vi "Stop Initiate RUN Procedure.vi"(8 "error in (no error)":errorcluster, 10 "Stop for good":bool, 11 "Tamer in":refnum<class "Tamer.lvclass">) -> (0 "error out":errorcluster, 3 "Tamer out":refnum<class "Tamer.lvclass">)   [LabVIEW 2020, in "TALOS.lvlib" / "Tamer.lvlib" / "Tamer.lvclass"]
uses:
  Tamer.lvclass
  C:/LabVIEW Code/TALOS/talos/Father of all uServices/Father of all uServices/Father of all uServices.lvclass
  Tamer.lvclass/Tamer.ctl
  Tamer Consumer Case Selector.ctl
  Guardian/Guardian/Requests.ctl
  Run Utilities/TypeDefs/Monkey Status.ctl
  Guardian/Guardian Messages/Requests from uServices Msg/Requests from uServices Msg.lvclass/Requests from uServices Msg.ctl
  Ancestor/Ancestor/Ancestor.lvclass/Ancestor.ctl
  Guardian/Guardian Messages/Requests from uServices Msg/Send Requests from uServices.vi
  Support VIs/Generate Error.vi
  FGV/Error Memory/Get Error Description.vi
  Support VIs/Get PC name.vi
  Ancestor/Ancestor/Read ID.vi
  Support VIs/Get Class Name.vi
  <vilib>/Utility/error.llb/Clear Errors.vi
  FGV/Error Memory/Error Memory Core.vi
  <vilib>/AdvancedString/Delimited String to 1D String Array.vi
  Support VIs/Circus Root Path.vi
  FGV/Error Memory/Error Crt Lvl checker.vi
  FGV/Error Memory/Error Memory Core.vi/40c8088d-b597-4017-91af-faa98e00292e.vi
  FGV/Error Memory/Error Memory Core.vi/d4a3ab98-063c-4e44-b43d-fbdcfe6c2be2.vi
  Father of all uServices/Father of all uServices/Father of all uServices.lvclass
  C:/LabVIEW Code/TALOS/builds/Actor Framework PPL/Actor Framework.lvlibp/1abvi3w/vi.lib/ActorFramework/Actor/Actor.lvclass
  builds/Actor Framework PPL/Actor Framework.lvlibp/1abvi3w/vi.lib/ActorFramework/Actor/Read Caller Enqueuer.vi
  builds/Actor Framework PPL/Actor Framework.lvlibp/1abvi3w/vi.lib/ActorFramework/Message Enqueuer/Enqueue.vi
  Support VIs/Global Memory.vi
  <vilib>/Utility/LVClass/Get LV Class Name.vi
  Support VIs/Is in Packed Library.vi
  Support VIs/TALOS Root path.vi
  Support VIs/Read CSV worksheet.vi
  Support VIs/Global Constants.vi
  <vilib>/Utility/error.llb/General Error Handler.vi
  Support VIs/Error Log.vi
  Guardian/Guardian Messages/Requests from uServices Msg/Requests from uServices Msg.lvclass
  Ancestor/Ancestor/Ancestor.lvclass
  <vilib>/Comparison/Equal/Equal Functor/Equal Functor.lvclass
  TALOS.lvlib
  Guardian/Guardian/Guardian.lvclass
  Run Utilities/Run Utilities.lvlib
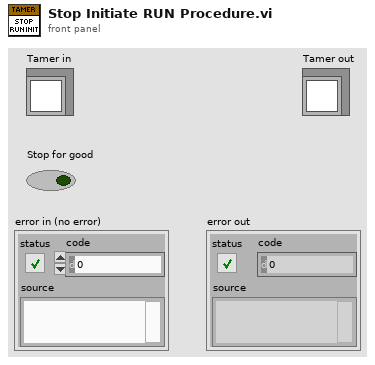
[diagram p1: front panel]
types:
  T1 = typedef "TALOS.lvlib/Tamer.lvlib/Tamer.lvclass/Tamer Consumer Case Selector.ctl" = enum16{"New schedule", "Initiate RUN", "Parse Schedules", "Script Checker", "Banana after Quality Check", "Update Crit Lvl", "Propagate Banana", "Reply from Guardian", "Reply from uService", "Timeout of RUN", "uService Replies Check", "Update from Monkey", "Monkey Died", "Reschedule", "Rerun", "Stop DAQ", "Stop Schedule", "Skip Run", "Kill Process", "Update GV"}
  T2 = typedef "TALOS.lvlib/Run Utilities.lvlib/Monkey Status.ctl" = enum16{"Init", "Paused", "Ongoing", "Stopped", "Finished (no errors)", "Finished (with errors)"}
  T3 = typedef "TALOS.lvlib/Guardian.lvlib/Guardian.lvclass/Requests.ctl" = enum16{"Ready to Launch", "Start RUN", "Stop RUN", "Update DAQ Params", "Update Error Listbox", "Update Run Status", "Update Kasli Log", "Run Stopped with Errors", "Switch uS View"}
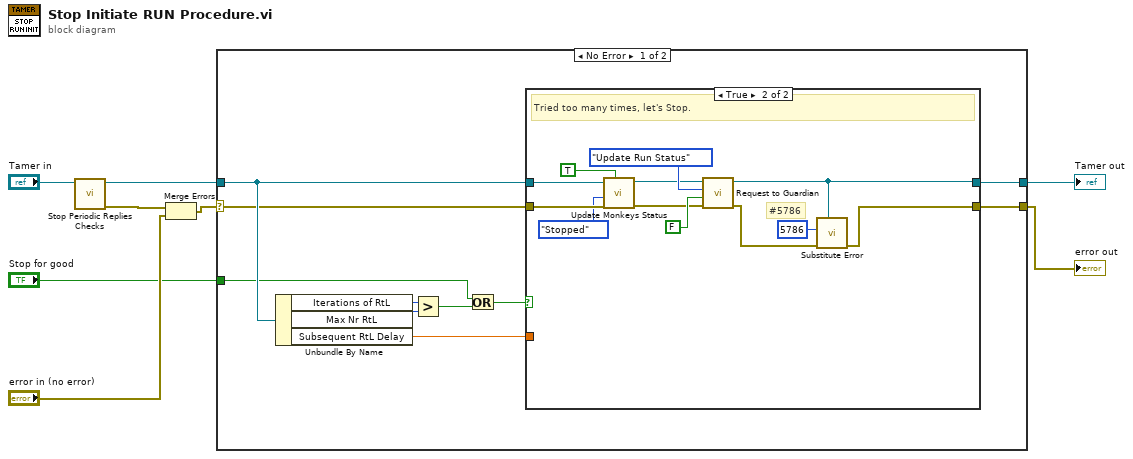
[diagram p0: block diagram]
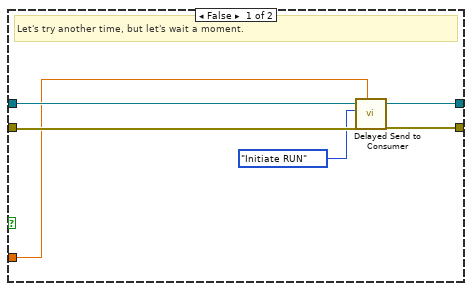
[diagram p2: hidden frame]
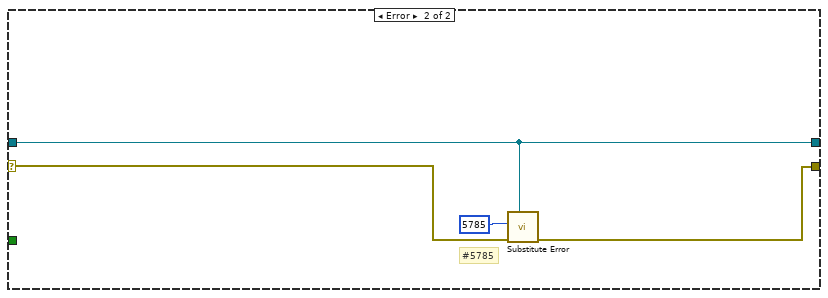
[diagram p3: hidden frame]
diagram:
  n1 = call-dynamic "Stop Periodic Replies Checks.vi"("Tamer in"="Tamer in") -> ("error out"=w2:errorcluster, "Tamer out"=w3:refnum<class "Tamer.lvclass">)  [unwired: 9 in]
  n2 = Merge Errors(w2, "error in (no error)") -> (w5:errorcluster)
  n3 = case shown="No Error" w5 {
    selector: w5 -> [w15 w37]
    tunnel: w3 -> [w17 w38]
    tunnel: [w16 w38] -> w6
    tunnel: [w14 w40] -> w8
    tunnel: "Stop for good" -> [w11 _]
    frame No Error {
      n4 = Unbundle By Name(w17) -> ("Iterations of RtL"=w18:u8, "Max Nr RtL"=w10:u8, "Subsequent RtL Delay"=w9:dbl)
      n5 = Greater?(x=w18, y=w10) -> (0:w13:bool)
      n6 = Or(x=w11, y=w13) -> (x .or. y?=w12:bool)
      n7 = case shown="True" w12 {
        tunnel: w17 -> [w24 w30]
        tunnel: [w23 w34] -> w16
        tunnel: w15 -> [w21 w28]
        tunnel: [w22 w36] -> w14
        tunnel: w9 -> [w20 _]
        frame False {
          # "Let's try another time, but let's wait a moment."
          n8 = call "Delayed Send to Consumer.vi"("Seconds (5)"=w20, "error in (no error)"=w21, "Case ID"=Tamer_Consumer_Case_Selector."Initiate RUN" ("Consumer Case Selector"), "Father of all uServices in"=w24) -> ("error out"=w22:errorcluster, "Father of all uServices out"=w23:refnum<class "Tamer.lvclass">)  [unwired: 6 in]
        }
        frame True {
          # "#5786"
          # "Tried too many times, let's Stop."
          n9 = call-dynamic "Update Monkeys Status.vi"("In ALL?"=TRUE, "error in (no error)"=w28, "Status"=Monkey_Status."Stopped", "Tamer in"=w30) -> ("error out"=w27:errorcluster, "Tamer out"=w29:refnum<class "Tamer.lvclass">)  [unwired: 6 in]
          n10 = call "Request to Guardian.vi"("error in (no error)"=w27, "Data"=FALSE, "Requests"=Requests."Update Run Status", "Father of all uServices in"=w29) -> ("error out"=w33:errorcluster, "Father of all uServices out"=w34:refnum<class "Tamer.lvclass">)  [unwired: 6 in]
          n11 = call "Substitute Error.vi"("LabVIEW Object"=w34, "error in (no error)"=w33, "Error Code"=5786) -> ("error out"=w36:errorcluster)  [unwired: 8 in]
        }
      }
    }
    frame Error {
      # "#5785"
      n12 = call "Substitute Error.vi"("LabVIEW Object"=w38, "error in (no error)"=w37, "Error Code"=5785) -> ("error out"=w40:errorcluster)  [unwired: 8 in]
    }
  }
  "error out" <- w8
  "Tamer out" <- w6
